vi "Reply Messaging.vi"() -> (3 "Pass?":bool)   [LabVIEW 2020, in "Messaging Tests.lvlib" / "Messaging Tests.lvclass"]
uses:
  Messaging Tests.lvclass
  Messaging Tests.lvclass/Messaging Tests.ctl
  Core/ActorFramework/Actor/Actor.lvclass
  TestActor/TestActor.lvclass
  Core/ActorFramework/Stop Msg/Stop Msg.lvclass
  Core/ActorFramework/LastAck/Last Ack.lvclass
  Core/ActorFramework/Reply Msg/Reply Msg.lvclass
  Divide Msg/Divide Msg.lvclass
  Increment2 Msg/Increment2 Msg.lvclass
  Core/ActorFramework/Message Queue/Message Queue.lvclass
  Core/ActorFramework/Message Dequeuer/Message Dequeuer.lvclass
  C:/Users/J63553/Projects/_LabVIEW Community/actor-framework/Core/ActorFramework/Message/Message.lvclass
  C:/Users/J63553/Projects/_LabVIEW Community/actor-framework/Core/ActorFramework/Reply Msg/Reply Msg.lvclass
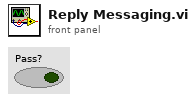
[diagram p1: front panel]
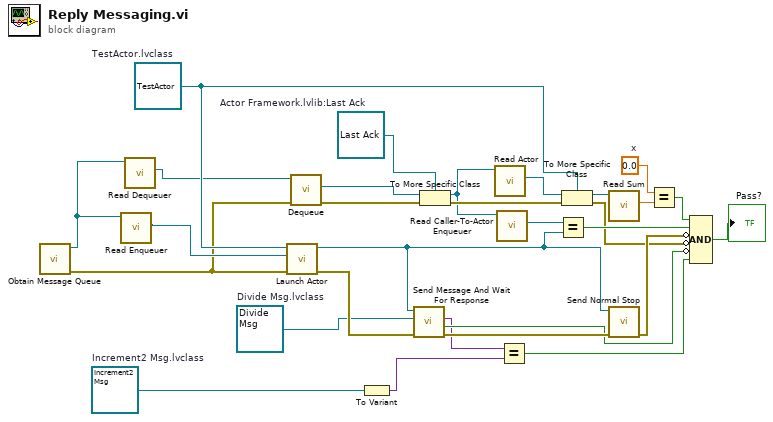
[diagram p0: block diagram]
diagram:
  w1 = refnum<class "Increment2 Msg.lvclass"> refnum  # Increment2 Msg.lvclass
  w12 = refnum<class "Divide Msg.lvclass"> refnum  # Divide Msg.lvclass
  w23 = 0.0  # x
  w29 = refnum<class "Last Ack.lvclass"> refnum  # Actor Framework.lvlib:Last Ack
  w26 = refnum<class "TestActor.lvclass"> refnum  # TestActor.lvclass
  n1 = call "Obtain Message Queue.vi"() -> ("error out"=w7:errorcluster, "Message Queue"=w10:refnum<class "Message Queue.lvclass">)  [unwired: 10 in]
  n2 = call "Read Enqueuer.vi"("Message Queue"=w10) -> ("Message Enqueuer"=w9:refnum<class "Message Enqueuer.lvclass">)  [unwired: 10 in]
  n3 = call "Read Dequeuer.vi"("Message Queue"=w10) -> ("Message Dequeuer"=w8:refnum<class "Message Dequeuer.lvclass">)  [unwired: 10 in]
  n4 = call "Launch Actor.vi"("error in (no error)"=w7, "Actor-to-Caller Enqueuer"=w9, "Actor"=w26) -> ("error out"=w15:errorcluster, "Caller-To-Actor Enqueuer"=w17:refnum<class "Message Enqueuer.lvclass">)  [unwired: 7 in]
  n5 = call "Dequeue.vi"("error in (no error)"=w7, "Message Dequeuer in"=w8) -> ("error out"=w6:errorcluster, "Message"=w5:refnum<class "Message.lvclass">)  [unwired: 5 in, 3 out]
  n6 = To Variant(anything=w1) -> (Variant=w2:variant)
  n7 = call "Send Message And Wait For Response.vi"("error in (no error)"=w15, "Original Message"=w12, "Message Enqueuer in"=w17) -> ("error out"=w16:errorcluster, "timed out?"=w14:bool, "Reply"=w11:variant)  [unwired: 5 in, 1 out]
  n8 = To More Specific Class(target class=w29, reference=w5, error in=w6) -> (specific class reference=w4:refnum<class "Last Ack.lvclass">, error out=w28:errorcluster)
  n9 = call "Read Actor.vi"("Last Ack"=w4) -> ("Actor"=w27:refnum<class "Actor.lvclass">)  [unwired: 10 in]
  n10 = call "Read Caller-To-Actor Enqueuer.vi"("Last Ack"=w4) -> ("Caller-to-Actor Enqueuer"=w3:refnum<class "Message Enqueuer.lvclass">)  [unwired: 10 in]
  n11 = Equal?(x=w11, y=w2) -> (x = y?=w13:bool)
  n12 = Equal?(x=w3, y=w17) -> (x = y?=w21:bool)
  n13 = To More Specific Class(target class=w26, reference=w27, error in=w28) -> (specific class reference=w25:refnum<class "TestActor.lvclass">, error out=w18:errorcluster)
  n14 = call "Read Sum.vi"("TestActor in"=w25) -> ("Sum"=w24:dbl)  [unwired: 9 in, 1 out]
  n15 = call "Send Normal Stop.vi"("error in (no error)"=w16, "Message Enqueuer"=w17) -> ("error out"=w19:errorcluster)  [unwired: 9 in]
  n16 = Equal?(x=w23, y=w24) -> (x = y?=w22:bool)
  n17 = Compound Arithmetic op=AND(w22, w21, invert w19, invert w18, invert w14, w13) -> (→"Pass?":bool)
